vi "Add Table to Today's Page.vi"(8 "Error In (No Error)":errorcluster, 9 "Delimiter":string=",", 10 "Notebook Name":string="My notebook on One Drive", 11 "User Email":string="myemail") -> (0 "error out":errorcluster, 2 "body":string, 3 "headers":string)   [LabVIEW 2019, in "OneNote Library.lvlib"]
uses:
  OneNote Library.lvlib
  c42b2f6f-2ce2-4546-a588-b289ee670433.vi
  <vilib>/JDP Science/JSONtext/Variant to JSON Text.vi
  Useful OAuth VIs/globals.vi
  <vilib>/httpClient/POSTBuffer.vi
  <vilib>/JDP Science/JSONtext/LVClass Serializer/JSONtext LVClass Serializer.lvclass
  <vilib>/httpClient/LabVIEWHTTPClient.lvlib
  Useful OAuth VIs/Useful OAuth VIs.lvlib
  Useful HTTP VIs/Useful HTTP VIs.lvlib
panel:
  out "Result":string
  out "Page ID":string
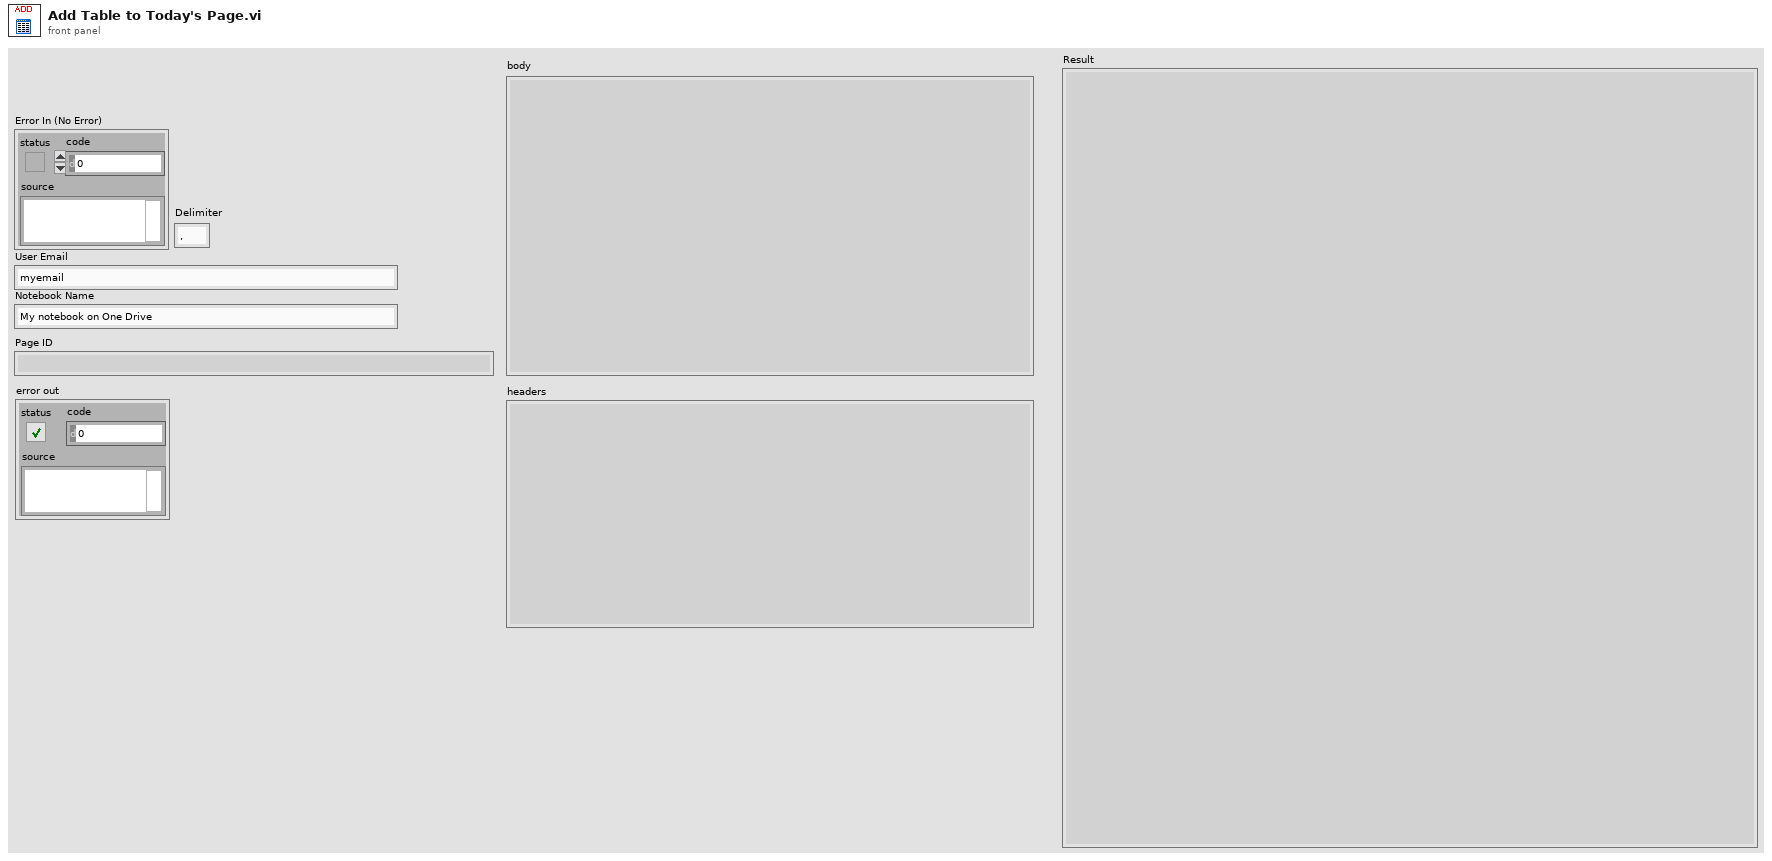
[diagram p1: front panel]
types:
  T1 = typedef "LabVIEWHTTPClient.lvlib/ClientHandle.ctl" = refnum<k1>
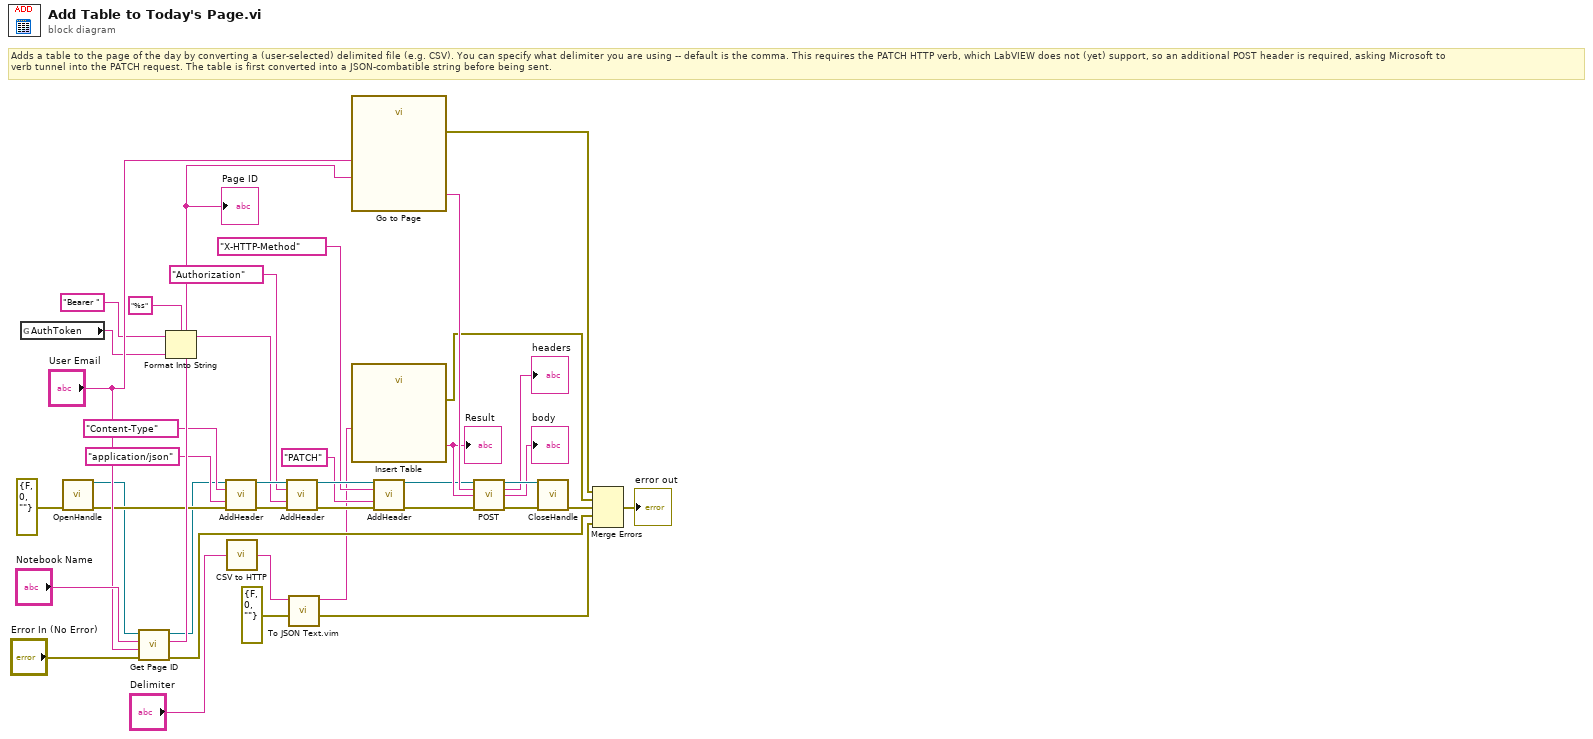
[diagram p0: block diagram]
diagram:
  # "Adds a table to the page of the day by converting a (user-selected) delimited file (e.g. CSV). You can specify what delimiter you are using -- default is the comma. This requires the PATCH HTTP verb, which LabVIEW does not (yet) support, so an additional POST header is required, asking Microsoft to \nverb tunnel into the PATCH request. The table is first converted into a JSON-combatible string before being sent."
  n1 = global read "globals.vi" "AuthToken"() -> (w26:string)
  n2 = call <vilib>:"OpenHandle.vi"("error in (no error)"=errorcluster {"status"=FALSE, "code"=0, "source"=""}) -> ("client handle out"=w16:T1, "error out"=w31:errorcluster)  [unwired: 13 in]
  n3 = call "Get Page ID.vi"("Error In (No Error)"="Error In (No Error)", "User Email"="User Email", "Notebook Name"="Notebook Name", "client handle"=w16) -> ("error out"=w17:errorcluster, "Page ID"=w36:string, "client handle out"=w15:T1)  [unwired: 5 in]
  "Page ID" <- w36
  n4 = Format Into String(format string="%s", initial string="Bearer ", w26) -> (resulting string=w27:string)  [unwired: 1 in, 1 out]
  n5 = call <vilib>:"AddHeader.vi"("client handle"=w15, "header"="Content-Type", "value"="application/json", "error in (no error)"=w31) -> ("client handle out"=w33:T1, "error out"=w32:errorcluster)  [unwired: 10 in]
  n6 = call "CSV to HTTP.vi"("Delimiter"="Delimiter") -> ("HTML Table"=w5:string)
  n7 = call <vilib>:"AddHeader.vi"("client handle"=w33, "header"="Authorization", "value"=w27, "error in (no error)"=w32) -> ("client handle out"=w12:T1, "error out"=w11:errorcluster)  [unwired: 10 in]
  n8 = call "To JSON Text.vim"("error in (no error)"=errorcluster {"status"=FALSE, "code"=0, "source"=""}, "Anything"=w5) -> ("error out"=w3:errorcluster, "<JSON>"=w4:string)  [unwired: 8 in]
  n9 = call "Go to Page"("user"="User Email", "Page ID"=w36) -> ("Result"=w25:string, "error out"=w21:errorcluster)  [unwired: 12 in]
  n10 = call "Insert Table"("Your Table Here"=w4) -> ("Result"=w24:string, "error out"=w20:errorcluster)  [unwired: 13 in]
  "Result" <- w24
  n11 = call <vilib>:"AddHeader.vi"("client handle"=w12, "header"="X-HTTP-Method", "value"="PATCH", "error in (no error)"=w11) -> ("client handle out"=w10:T1, "error out"=w9:errorcluster)  [unwired: 10 in]
  n12 = call-poly <vilib>:"POST.vi"("client handle"=w10, "url"=w25, "buffer"=w24, "error in (no error)"=w9) -> ("client handle out"=w23:T1, "headers"=→"headers":string, "body"=→"body":string, "error out"=w22:errorcluster)  [unwired: 8 in]
  n13 = call <vilib>:"CloseHandle.vi"("client handle"=w23, "error in (no error)"=w22) -> ("error out"=w19:errorcluster)  [unwired: 13 in]
  n14 = Merge Errors(w21, w20, w19, w17, w3) -> (→"error out":errorcluster)
